vi "Pkt - Check Packet Type.vi"(8 "error in (no error)":errorcluster, 11 "Node Ptr In":T2 format="%.0x") -> (0 "error out":errorcluster, 2 "Packet Type":T1, 3 "Node Ptr Out":T2 format="%.0x")   [LabVIEW 2019, in "UDP-Custom-Device System Explorer.lvlib"]
uses:
  UDP-Custom-Device System Explorer.lvlib
  <vilib>/NI VeriStand/Custom Device API/Custom Device Item Ref.ctl
  Types/Packet Info/Packet Type.ctl
  Shared/Constants.vi
  Shared/UDP-Custom-Device Shared.lvlib
  <vilib>/NI VeriStand/Custom Device API/Custom Device API.lvlib
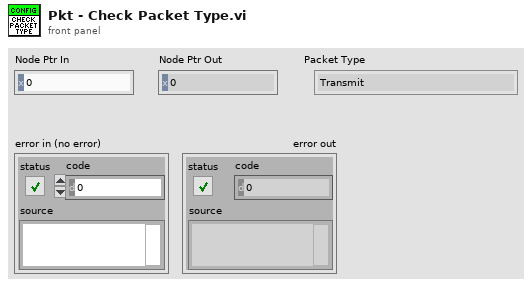
[diagram p1: front panel]
types:
  T1 = typedef "UDP-Custom-Device System Explorer.lvlib/Packet Type.ctl" = enum16{"Transmit", "Receive", "Buffered Transmit", "Buffered Receive"}
  T2 = typedef "Custom Device API.lvlib/Custom Device Item Ref.ctl" = u64
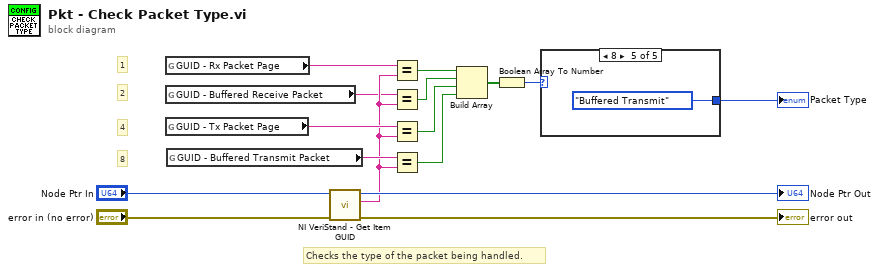
[diagram p0: block diagram]
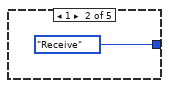
[diagram p3: hidden frame]
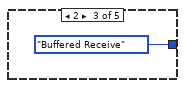
[diagram p4: hidden frame]
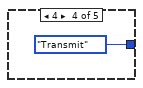
[diagram p5: hidden frame]
diagram:
  # "8"
  # "4"
  # "2"
  # "1"
  # "Checks the type of the packet being handled."
  n1 = global read "Constants.vi" "GUID - Rx Packet Page"() -> (w2:string)
  n2 = global read "Constants.vi" "GUID - Buffered Receive Packet"() -> (w1:string)
  n3 = global read "Constants.vi" "GUID - Tx Packet Page"() -> (w4:string)
  n4 = global read "Constants.vi" "GUID - Buffered Transmit Packet"() -> (w5:string)
  n5 = call <vilib>:"NI VeriStand - Get Item GUID.vi"("error in (no error)"="error in (no error)", "Item Ref in"="Node Ptr In") -> ("error out"=→"error out":errorcluster, "GUID"=w3:string, "Item Ref out"=→"Node Ptr Out":T2)  [unwired: 7 in]
  n6 = Equal?(x=w2, y=w3) -> (x = y?=w12:bool)
  n7 = Equal?(x=w1, y=w3) -> (x = y?=w11:bool)
  n8 = Equal?(x=w4, y=w3) -> (x = y?=w10:bool)
  n9 = Equal?(x=w5, y=w3) -> (x = y?=w9:bool)
  n10 = Build Array(w12, w11, w10, w9) -> (w8:bool[])
  n11 = Boolean Array To Number(Boolean array=w8) -> (number=w7:u32)
  n12 = case shown="8" w7 {
    tunnel: [_ Packet_Type."Receive" ("Packet Type") Packet_Type."Buffered Receive" ("Packet Type") Packet_Type."Transmit" ("Packet Type") Packet_Type."Buffered Transmit" ("Packet Type")] -> w6
    frame 0, Default {
    }
    frame 1 {
    }
    frame 2 {
    }
    frame 4 {
    }
    frame 8 {
    }
  }
  "Packet Type" <- w6
